vi "read all lines.vi"(8 "error in (no error)":errorcluster, 11 "Arduino Uno in":refnum<class "Arduino Uno.lvclass">) -> (0 "error out":errorcluster, 2 "Array":dbl[](array[numeric]), 3 "Arduino Uno out":refnum<class "Arduino Uno.lvclass">)   [LabVIEW 2025, in "USB IO.lvlib" / "Arduino Uno.lvclass"]
uses:
  Arduino Uno.lvclass
  Arduino Uno.lvclass/Arduino Uno.ctl
  <vilib>/MakerHub/LINX/Public/Peripherals/Analog/Analog Read 1 Chan.vi
  <vilib>/MakerHub/LINX/Public/Peripherals/Analog/Analog Read N Chans.vi
  <vilib>/MakerHub/LINX/Private/Local IO/LinxAnalogRead.vi
  <vilib>/MakerHub/LINX/Public/Utilities/Check Channel.vi
  <vilib>/MakerHub/LINX/Private/Utilties/Generate Error.vi
  <vilib>/MakerHub/LINX/LMH-LINX.lvlib
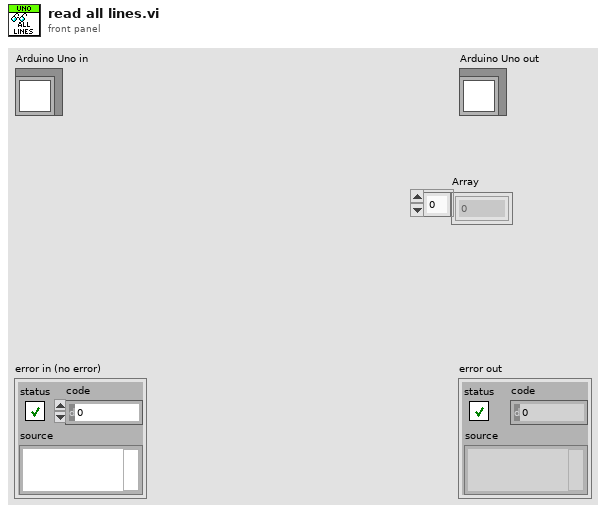
[diagram p1: front panel]
types:
  T1 = typedef "LMH-LINX.lvlib/LINX Ref.ctl" = cluster{"IO":T2, "Interface":T3, "LINX Device Config":T4}
  T2 = typedef "LMH-LINX.lvlib/Platform.ctl" = enum16{"Remote", "Local"}
  T3 = typedef "LMH-LINX.lvlib/Interface.ctl" = enum16{"Serial", "TCP"}
  T4 = typedef "LMH-LINX.lvlib/Device.lvlib/LINX Device Config.ctl" = cluster{"Interface":T3, "COM Port":refnum<visa-resource-name>, "TCP Configuration":T5, "Device Family":u8, "Device ID":u8, "Device Name":string, "TCP Ref":refnum<k5>, "Channels":T6}
  T5 = typedef "LMH-LINX.lvlib/Device.lvlib/TCP Config.ctl" = cluster{"IP Address":string, "Port":u16}
  T6 = typedef "LMH-LINX.lvlib/Channels.ctl" = cluster{"DI":u8[], "DO":u8[], "AI":u8[], "AO":u8[], "PWM":u8[], "QE":u8[], "UART":u8[], "I2C 2":u8[], "SPI":u8[], "CAN":u8[], "Servo":u8[], "AI Ref (V)":dbl, "AI Resolution (Bits)":u8, "AO Ref (V)":dbl, "AO Resolution (Bits)":u8}
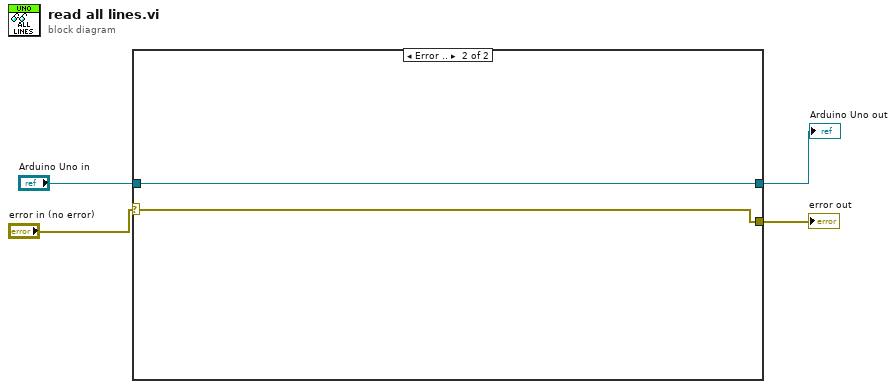
[diagram p0: block diagram]
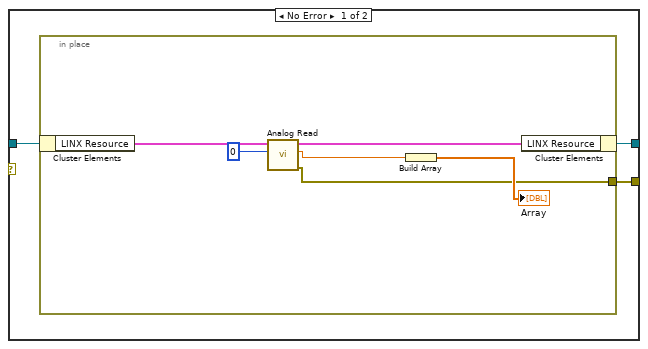
[diagram p2: hidden frame]
diagram:
  n1 = case shown="Error .." "error in (no error)" {
    selector: "error in (no error)" -> [_ w14]
    tunnel: "Arduino Uno in" -> [w7 w15]
    tunnel: [w6 w15] -> w2
    tunnel: [w5 w14] -> w1
    frame No Error {
      n2 = in-place {
        in-place-border: [w8] -> w5
        n3 = in-place-cluster #1(w7) -> ("LINX Resource"=w13:T1)
        n4 = call-poly <vilib>:"Analog Read.vi"("Analog Channel"=u8 0, "LINX Resource"=w13) -> ("Error Out"=w8:errorcluster, "Voltage"=w10:dbl, "LINX Resource"=w12:T1)  [unwired: 6 in, 1 out]
        n5 = Build Array(w10) -> (→"Array":dbl[])
        n6 = in-place-cluster #1("LINX Resource"=w12) -> (w6:refnum<class "Arduino Uno.lvclass">)
      }
    }
    frame Error {
    }
  }
  "error out" <- w1
  "Arduino Uno out" <- w2
